vi "Deadzone.vi"(1 "valDeadzone":dbl, 2 "valInput":dbl) -> (0 "valOutput":dbl)   [LabVIEW 2018]
doc: "Test input to see if absolute value is GEQ 0.1\nIf TRUE, invert and send out ELSE send zero"
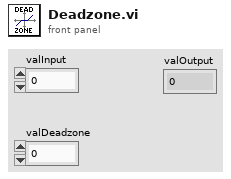
[diagram p1: front panel]
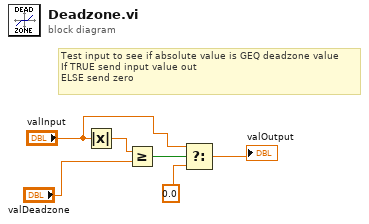
[diagram p0: block diagram]
diagram:
  # "Test input to see if absolute value is GEQ deadzone value\nIf TRUE send input value out \nELSE send zero"
  n1 = Absolute Value(x="valInput") -> (abs(x)=w6:dbl)
  n2 = Greater Or Equal?(x=w6, y="valDeadzone") -> (x >= y?=w5:bool)
  n3 = Select(t="valInput", s=w5, f=0.0) -> (s? t:f=→"valOutput":dbl)
